vi "verify_files.vi"(8 "error in (no error)":errorcluster, 10 "File or Directory":path) -> (0 "error out":errorcluster, 2 "Array":path[](array[path]))   [LabVIEW 2010, in "ErrorController.lvclass"]
uses:
  ErrorController.lvclass
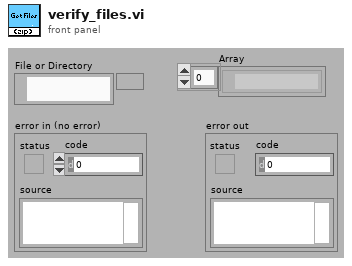
[diagram p1: front panel]
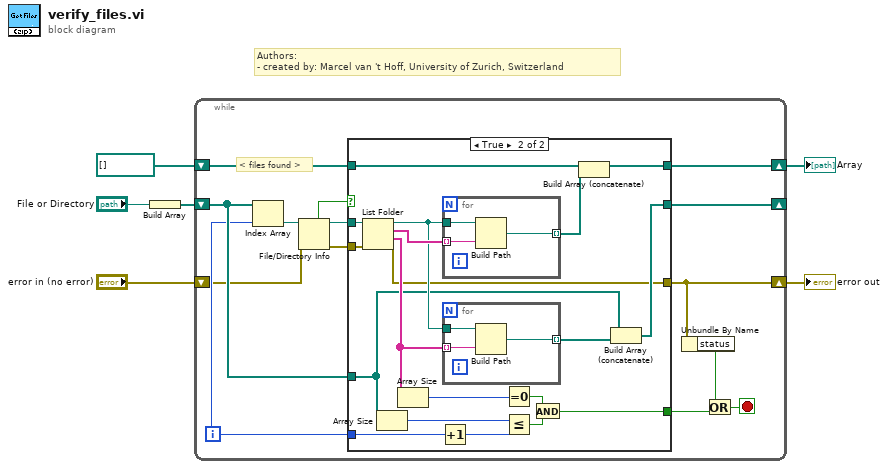
[diagram p0: block diagram]
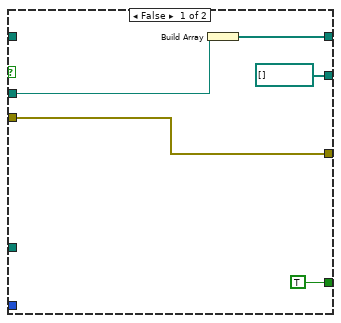
[diagram p2: hidden frame]
diagram:
  # "Authors: \n- created by: Marcel van 't Hoff, University of Zurich, Switzerland"
  n1 = Build Array("File or Directory") -> (w3:path[])
  n2 = while {
    shift-right: [w20] -> _
    shift-left: w3 -> [w19]
    shift-right: [w18] -> w5
    shift-left: path[] [] -> [w17]
    shift-right: [w10] -> w1
    shift-left: "error in (no error)" -> [w12]
    i -> [w13]
    stop <- w9 stop-if-true
    # "< files found >"
    n3 = Index Array(array=w19, index=w13) -> (element=w16:path)
    n4 = File/Directory Info(path=w16, error in=w12) -> (path out=w14:path, directory=w15:bool, error out=w11:errorcluster)  [unwired: 4 out]
    n5 = case shown="True" w15 {
      tunnel: w14 -> [w22 w44]
      tunnel: [path[] [] w41] -> w20
      tunnel: w19 -> [_ w34]
      tunnel: [w23 w38] -> w18
      tunnel: w17 -> [_ w37]
      tunnel: [TRUE w30] -> w8
      tunnel: w13 -> [_ w28]
      tunnel: w11 -> [w21 w27]
      tunnel: [w21 w26] -> w10
      frame False {
        n6 = Build Array(w22) -> (w23:path[])
      }
      frame True {
        n7 = List Folder(path=w44, error in=w27) -> (path out=w42:path, filenames=w43:string[], folder names=w35:string[], error out=w26:errorcluster)  [unwired: 2 out]
        n8 = Array Size(array=w34) -> (size(s)=w33:i32)
        n9 = Array Size(array=w35) -> (size(s)=w36:i32)
        n10 = Increment(x=w28) -> (x+1=w29:i32)
        n11 = for {
          tunnel: w42 -> [w50]
          tunnel: w43 -> [w49] mode=indexing
          tunnel: [w48] -> w39 mode=indexing
          n12 = Build Path(base path=w50, name or relative path=w49) -> (appended path=w48:path)
        }
        n13 = for {
          tunnel: w42 -> [w47]
          tunnel: w35 -> [w46] mode=indexing
          tunnel: [w45] -> w40 mode=indexing
          n14 = Build Path(base path=w47, name or relative path=w46) -> (appended path=w45:path)
        }
        n15 = Equal To 0?(x=w36) -> (x = 0?=w32:bool)
        n16 = Less Or Equal?(x=w33, y=w29) -> (x <= y?=w31:bool)
        n17 = And(x=w32, y=w31) -> (x .and. y?=w30:bool)
        n18 = Build Array (concatenate)(w37, w39) -> (w38:path[])
        n19 = Build Array (concatenate)(w34, w40) -> (w41:path[])
      }
    }
    n20 = Unbundle By Name(w10) -> ("status"=w7:bool)
    n21 = Or(x=w7, y=w8) -> (x .or. y?=w9:bool)
  }
  "Array" <- w5
  "error out" <- w1
